vi "Compose Cluster - Mixed - Element Value.vi"() -> ()   [LabVIEW 2017, in "Composition.Tests.lvlib"]
uses:
  Composition.Tests.lvlib
  f9f3226b-254d-4f9f-8b82-83f2d79073c2.vi
  <vilib>/addons/_JKI Toolkits/Caraya/classes/Test/Test.lvclass
  <vilib>/addons/_JKI Toolkits/Caraya/classes/Assert/Assert.lvclass
panel:
  out "error out":errorcluster
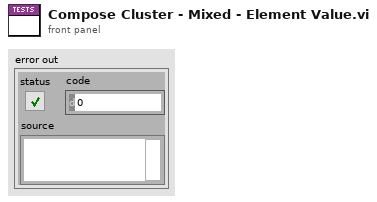
[diagram p1: front panel]
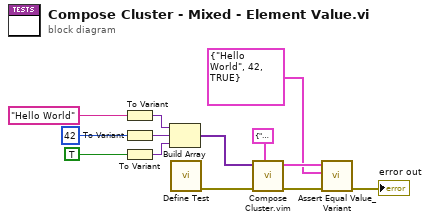
[diagram p0: block diagram]
diagram:
  n1 = To Variant(anything="Hello World") -> (Variant=w8:variant)
  n2 = To Variant(anything=42) -> (Variant=w9:variant)
  n3 = To Variant(anything=TRUE) -> (Variant=w10:variant)
  n4 = Build Array(w8, w9, w10) -> (w7:variant[])
  n5 = call <vilib>:"Define Test.vi"() -> ("error out"=w3:errorcluster)  [unwired: 11 in]
  n6 = call "Compose Cluster.vim"("Type"=cluster{string, i32, bool} {"", 0, FALSE}, "error in"=w3, "Elements"=w7) -> ("error out"=w5:errorcluster, "Cluster"=w2:cluster{string, i32, bool})  [unwired: 7 in]
  n7 = call <vilib>:"Assert Equal Value_Variant.vi"("error in (no error)"=w5, "Y"=cluster{string, i32, bool} {"Hello World", 42, TRUE}, "X"=w2) -> ("error out"=→"error out":errorcluster)  [unwired: 8 in]
